vi "post_artifacts.vi"(8 "error in (no error)":errorcluster, 10 "build_spec_info [] in":T1[](array[typedef]), 11 "lv-builder in":refnum<class "lv-builder.lvclass">) -> (0 "error out":errorcluster, 2 "build_spec_info [] out":T1[](array[typedef]), 3 "lv-builder out":refnum<class "lv-builder.lvclass">)   [LabVIEW 2015, in "lv-builder.lvclass"]
uses:
  lv-builder.lvclass
  lv-build/public/_controls/build_specification.ctl
  lv-build/public/_controls/build_type.ctl
  lv-build/lv-build.lvlib
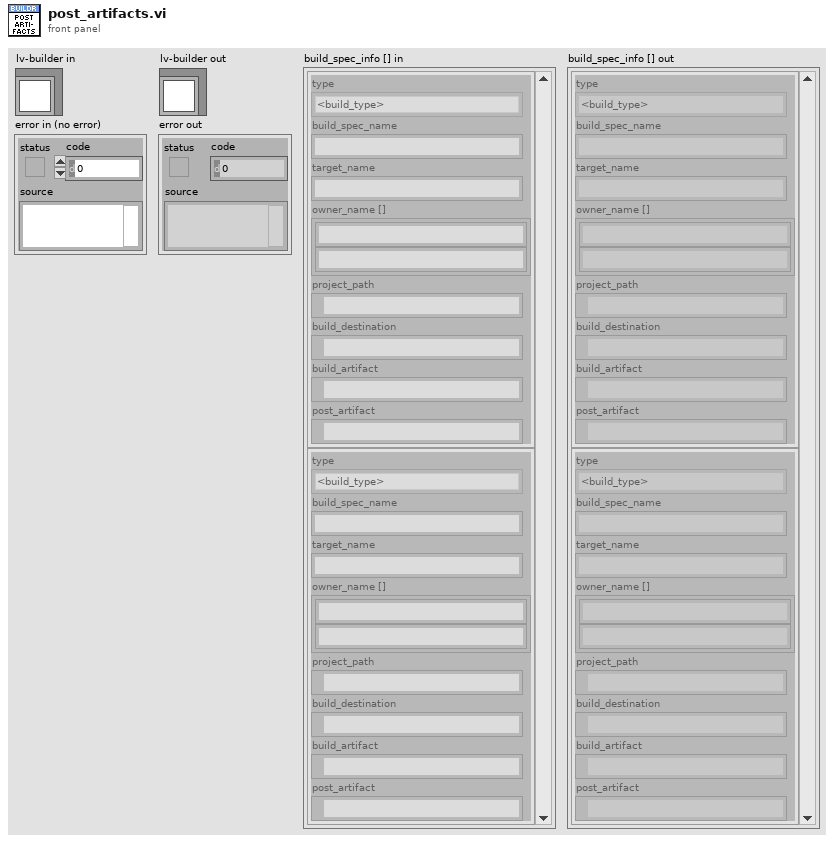
[diagram p1: front panel]
types:
  T1 = typedef "lv-build.lvlib/build_specification.ctl" = cluster{"type":T2, "build_spec_name":string, "target_name":string, "owner_name []":string[], "project_path":path, "build_destination":path, "build_artifact":path, "post_artifact":path}
  T2 = typedef "lv-build.lvlib/build_type.ctl" = enum16{"<build_type>", "application_pc", "application_rt", "installer", "llb", "lvlibp", "zip", "fpga", "<null>"}
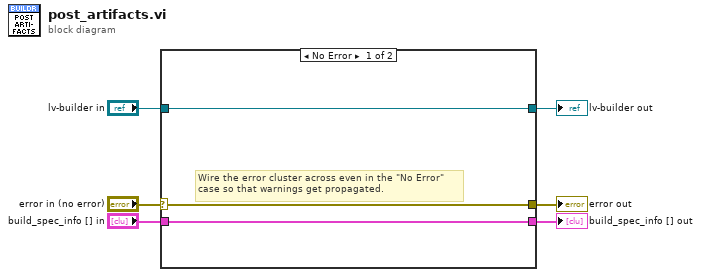
[diagram p0: block diagram]
diagram:
  n1 = case shown="No Error" "error in (no error)" {
    selector: "error in (no error)" -> [w8 w12]
    tunnel: [w8 w12] -> w5
    tunnel: [w9 w11] -> w3
    tunnel: "lv-builder in" -> [w9 w11]
    tunnel: "build_spec_info [] in" -> [w7 w10]
    tunnel: [w7 w10] -> w1
    frame No Error {
      # "Wire the error cluster across even in the \"No Error\"\ncase so that warnings get propagated."
    }
    frame Error {
    }
  }
  "error out" <- w5
  "lv-builder out" <- w3
  "build_spec_info [] out" <- w1
